vi "HDF5 Test.vi"() -> ()   [LabVIEW 2019]
uses:
  HDF5 Tools.lvlib
panel:
  in  "My Cluster 2":T1
  in  "My Cluster":T1
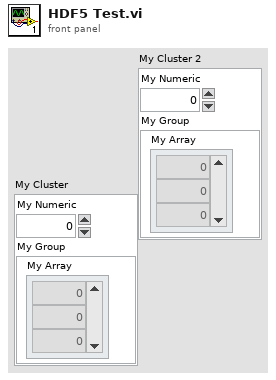
[diagram p1: front panel]
types:
  T1 = cluster{"My Numeric":dbl, "My Group":cluster{"My Array":dbl[]}}
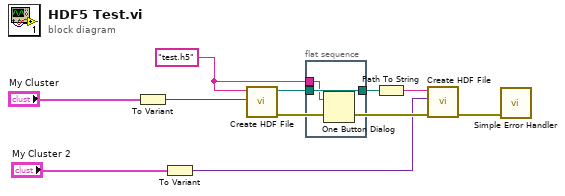
[diagram p0: block diagram]
diagram:
  w1 = "test.h5" ("path")
  n1 = To Variant(anything="My Cluster") -> (Variant=w10:variant)
  n2 = To Variant(anything="My Cluster 2") -> (Variant=w4:variant)
  n3 = call "Create HDF File.vi"("variant"=w10, "path"=w1) -> ("error out"=w8:errorcluster, "path out"=w3:path)  [unwired: 7 in, 1 out]
  n4 = flat-sequence {
    tunnel: w3 -> [w12]
    tunnel: [w12] -> w2
    tunnel: w1 -> [w11]
    frame #0 {
      n5 = One Button Dialog(message=w11) -> ()  [unwired: 1 in, 1 out]
    }
  }
  n6 = Path To String(path=w2) -> (string=w5:string)
  n7 = call "Create HDF File.vi"("error in (no error)"=w8, "variant"=w4, "path"=w5) -> ("error out"=w7:errorcluster)  [unwired: 6 in, 2 out]
  n8 = call <vilib>:"Simple Error Handler.vi"("error in (no error)"=w7) -> ()  [unwired: 4 in, 5 out]
